vi "Get all Queue.vi"(8 "error in (no error)":errorcluster, 11 "uService List":refnum<class "uService List.lvclass">) -> (0 "error out":errorcluster, 2 "All queues":refnum<class "Message Enqueuer.lvclass">[](array[class]), 3 "uService List out":refnum<class "uService List.lvclass">)   [LabVIEW 2026, in "TALOS.lvlib" / "Classes.lvlib" / "uService List.lvclass"]
uses:
  uService List.lvclass
  builds/Actor Framework PPL/Actor Framework.lvlibp/1abvi3w/vi.lib/ActorFramework/Message Enqueuer/Message Enqueuer.lvclass
  uService List.lvclass/uService List.ctl
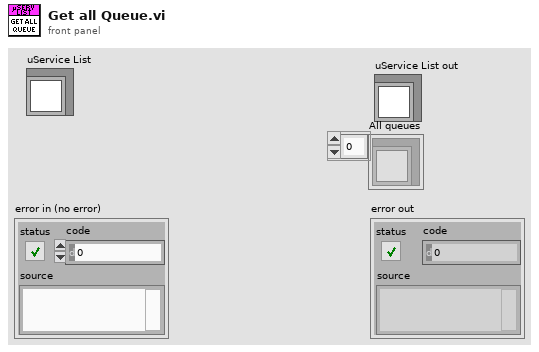
[diagram p1: front panel]
types:
  T1 = typedef "TALOS.lvlib/Classes.lvlib/uService List.lvclass/uService Properties.ctl" = cluster{"uService Queue":refnum<class "Message Enqueuer.lvclass">, "Last Pat":timestamp, "Online":bool, "Vi Ref":refnum<vi>, "Class name":string, "GUI":bool, "FP Items Refs Map":map{string, refnum<vi>}, "Remote GUI":bool, "Remote Window":refnum<vi>}
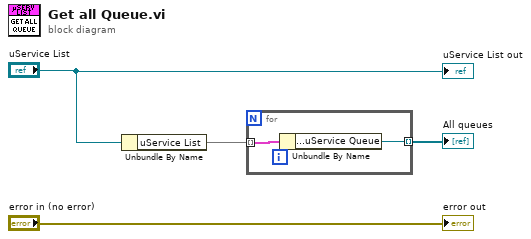
[diagram p0: block diagram]
diagram:
  n1 = Unbundle By Name("uService List") -> ("uService List"=w4:map{string, T1})
  n2 = for {
    tunnel: w4 -> [w6] mode=indexing
    tunnel: [w5] -> w1 mode=indexing
    n3 = Unbundle By Name(w6) -> ("uService Properties.uService Queue"=w5:refnum<class "Message Enqueuer.lvclass">)
  }
  "All queues" <- w1
  "error out" <- "error in (no error)"
  "uService List out" <- "uService List"
